vi "CSGaussmeter.setRelvalue.vi"(0 "i ref in":refnum<vi>, 7 "Relative value":dbl, 9 "Unit":T1, 11 "error in (no error)":errorcluster) -> (4 "i ref out":refnum<vi>, 15 "error out":errorcluster)   [LabVIEW 2014, in "CSGaussmeter.lvlib"]
doc: "Dieses VI setzt den Bezugswert für die Relative-Funktion\n\n\nThis VI sets the reference value for the Relative function"
uses:
  CSGaussmeter.lvlib
  instr.lib/FH_55/TypeDef/Unit2.ctl
  CS_Core/CSObj/CSObj.lvlib
  CSlibraries/UtilityLib/UtilityLib.lvlib
  instr.lib/FH_55/FH 55.lvlib
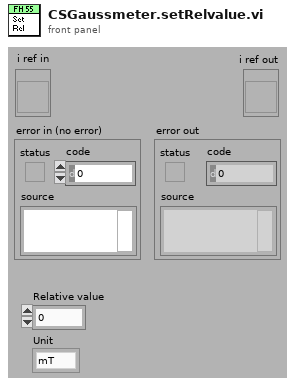
[diagram p1: front panel]
types:
  T1 = typedef "FH 55.lvlib/Unit2.ctl" = enum16{"mT", "G", "kA/m"}
  T2 = typedef "CSGaussmeter.lvlib/CSGaussmeter.i attribute.ctl" = cluster{"Name":string, "VISA Resource Name":refnum<visa-resource-name>, "actValues":cluster{" Limit":bool, "Unit ":T3, "Temp_Unit":T4, "Max":T5, " Filter":bool, " Peak":bool, " Auto_Range":bool, "Range":T6, " Rel":bool, " CTemp":bool, " CField":bool, "AC_DC ":bool, "Set_lower":cluster{"Numeric":dbl, "Cancel Button":bool, "Unit":T1}, "Set_upper":cluster{"Numeric":dbl, "Cancel Button":bool, "Unit":T1}, "Set_Rel":cluster{"Numeric":dbl, "Cancel Button":bool, "Unit":T1}, "Zero":bool, " Local":bool, "Reset":bool, " Init":bool}, "FH 55 Gauss-/Teslameter":T7, "MAX_Value":T8, "MIN_Value":T8, "Rel_Value":T8, "Array ":string[], "LIMU":dbl, " LIML":dbl, "Messwerte 2":string, "Messwerte ":cluster{"Numeric":i32, "OK Button":bool}, "serviceID":cluster{"Current ID":i32, "Unit ID":i32, "Temp ID":i32, "Name ID \n":i32, "Visa ID ":i32}, "setValues ":cluster{" Limit":bool, "Unit ":T3, "Temp_Unit":T4, "Max":T5, " Filter":bool, " Peak":bool, " Auto_Range":bool, "Range":T6, " Rel":bool, " CTemp":bool, " CField":bool, "AC_DC ":bool, "Set_lower":cluster{"Numeric":dbl, "Cancel Button":bool, "Unit":T1}, "Set_upper":cluster{"Numeric":dbl, "Cancel Button":bool, "Unit":T1}, "Set_Rel":cluster{"Numeric":dbl, "Cancel Button":bool, "Unit":T1}, "Zero":bool, " Local":bool, "Reset":bool, " Init":bool}}
  T3 = typedef "FH 55.lvlib/Unit.ctl" = enum16{"T", "G", "A/m"}
  T4 = typedef "FH 55.lvlib/Temp_Unit.ctl" = enum16{"Temp off", "Celsius", "Fahrenheit"}
  T5 = typedef "FH 55.lvlib/Max.ctl" = enum16{"MAX off", "Show MAX", "MAX/MIN"}
  T6 = typedef "FH 55.lvlib/Range.ctl" = enum16{"1", "2", "3", "4", "5", "6", "7"}
  T7 = typedef "FH 55.lvlib/Display.ctl" = cluster{"current value":string, "Limit":string, "Remote":string, "function ":string, "Cluster":cluster{"AC/DC":string, "Auto":string, "Filter":string, "Range":string, "Rel":string, "Peak":string}}
  T8 = typedef "FH 55.lvlib/Value_String.ctl" = cluster{"Numeric":dbl, "String":string}
  T9 = cluster{"Numeric":dbl, "Cancel Button":bool, "Unit":T1}
  T10 = cluster{"VISA Resource Name":refnum<visa-resource-name>}
  T11 = typedef "FH 55.lvlib/VisaCluster.ctl" = cluster{"VISA Resource Name":refnum<visa-resource-name>}
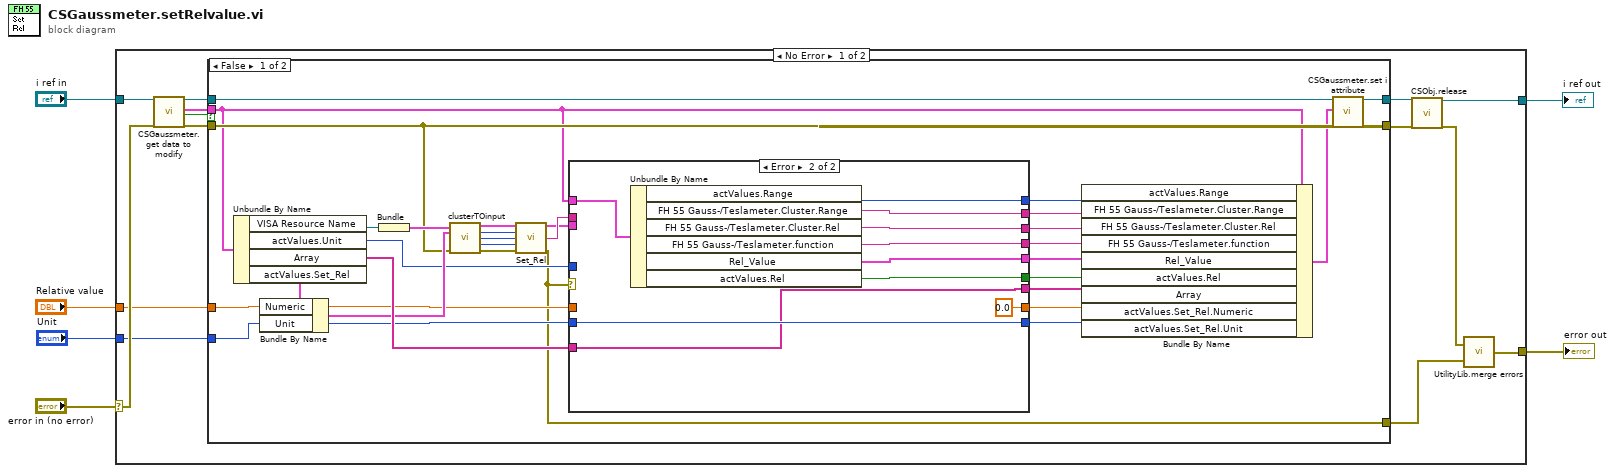
[diagram p0: block diagram]
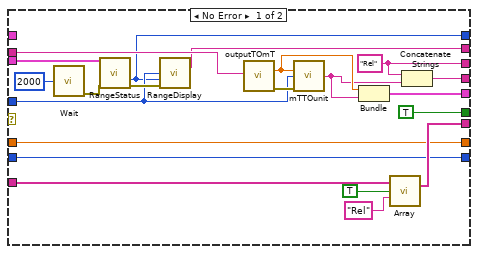
[diagram p2: hidden frame]
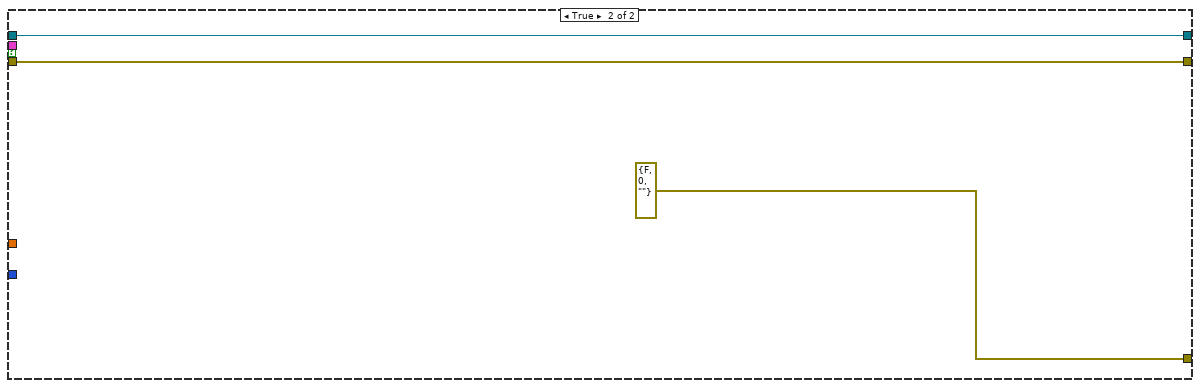
[diagram p3: hidden frame]
diagram:
  n1 = case shown="No Error" "error in (no error)" {
    selector: "error in (no error)" -> [w15 w84]
    tunnel: [w16 w84] -> w3
    tunnel: "i ref in" -> [w14 w85]
    tunnel: [w7 w85] -> w4
    tunnel: "Relative value" -> [w8 _]
    tunnel: "Unit" -> [w9 _]
    frame No Error {
      n2 = call "CSGaussmeter.get data to modify.vi"("i ref in"=w14, "error in (no error)"=w15) -> ("i ref out"=w13:refnum<vi>, "i attribute"=w12:T2, "timed out"=w11:bool, "error out"=w10:errorcluster)  [unwired: 14 in]
      n3 = case shown="False" w11 {
        tunnel: w13 -> [w48 w82]
        tunnel: w10 -> [w32 w83]
        tunnel: w12 -> [w21 _]
        tunnel: [w32 w83] -> w18
        tunnel: [w47 w82] -> w20
        tunnel: [w24 errorcluster {"status"=FALSE, "code"=0, "source"=""} ("error out")] -> w17
        tunnel: w9 -> [w25 _]
        tunnel: w8 -> [w26 _]
        frame False {
          n4 = Unbundle By Name(w21) -> ("VISA Resource Name"=w49:refnum<visa-resource-name>, "actValues.Unit"=w29:T3, "Array"=w39:string[], "actValues.Set_Rel"=w31:T9)
          n5 = Bundle By Name(cluster=w31, "Numeric"=w26, "Unit"=w25) -> (w34:T9)
          n6 = Bundle("VISA Resource Name"=w49) -> (w46:T10)  [unwired: 1 in]
          n7 = call "clusterTOinput.vi"("Set_Rel"=w34, "error in (no error)"=w32) -> ("Range"=w35:T6, "Numeric"=w36:i32, "Unit"=w37:T3, "error out"=w33:errorcluster)  [unwired: 10 in]
          n8 = call "Set_Rel.vi"("VisaCluster"=w46, "Range"=w35, "Numeric"=w36, "Unit"=w37, "error in (no error)"=w33) -> ("VisaCluster"=w30:T11, "Answer"=w43:string, "error out"=w24:errorcluster)  [unwired: 8 in]
          n9 = case shown="Error" w24 {
            tunnel: [TRUE ("actValues.Rel") w72] -> w44
            tunnel: w43 -> [w69 _]
            tunnel: [w68 w74] -> w42
            tunnel: [w67 w73] -> w41
            tunnel: [w66 w71] -> w40
            tunnel: w39 -> [w61 w78]
            tunnel: [w60 w78] -> w38
            tunnel: w30 -> [w58 _]
            tunnel: w29 -> [w56 _]
            tunnel: [w55 w75] -> w28
            tunnel: [w54 w76] -> w27
            tunnel: w26 -> [w53 _]
            tunnel: w25 -> [w52 w80]
            tunnel: [w53 0.0 ("Numeric")] -> w23
            tunnel: [w52 w80] -> w22
            tunnel: w21 -> [_ w77]
            frame No Error {
              w68 = "Rel" ("FH 55 Gauss-/Teslameter.Cluster.Rel")
              n10 = call "Wait.vi"("milliseconds to wait"=u32 2000) -> ("error out"=w51:errorcluster)  [unwired: 14 in]
              n11 = call "RangeStatus.vi"("VisaCluster"=w58, "error in (no error)"=w51) -> ("Range"=w54:T6, "error out"=w57:errorcluster)  [unwired: 10 in, 2 out]
              n12 = call "RangeDisplay.vi"("Unit"=w56, "Range"=w54, "error in (no error)"=w57) -> ("Display"=w55:string)  [unwired: 10 in, 2 out]
              n13 = call "outputTOmT.vi"("Input"=w69) -> ("Numeric"=w65:dbl, "error out"=w59:errorcluster)  [unwired: 13 in]
              n14 = call "mTTOunit.vi"("Numeric"=w65, "Unit"=w56, "error in (no error)"=w59) -> ("Display"=w64:string)  [unwired: 10 in, 2 out]
              n15 = Bundle("Numeric"=w65, "Display"=w64) -> (w66:cluster{"Numeric":dbl, "Display":string})  [unwired: 1 in]
              n16 = call "Array.vi"("Array"=w61, "Boolean"=TRUE, "String"="Rel" ("element")) -> ("Array"=w60:string[])  [unwired: 12 in]
              n17 = Concatenate Strings(w68, w64) -> (w67:string)
            }
            frame Error {
              n18 = Unbundle By Name(w77) -> ("actValues.Range"=w76:T6, "FH 55 Gauss-/Teslameter.Cluster.Range"=w75:string, "FH 55 Gauss-/Teslameter.Cluster.Rel"=w74:string, "FH 55 Gauss-/Teslameter.function"=w73:string, "Rel_Value"=w71:T8, "actValues.Rel"=w72:bool)
            }
          }
          n19 = Bundle By Name(cluster=w21, "actValues.Range"=w27, "FH 55 Gauss-/Teslameter.Cluster.Range"=w28, "FH 55 Gauss-/Teslameter.Cluster.Rel"=w42, "FH 55 Gauss-/Teslameter.function"=w41, "Rel_Value"=w40, "actValues.Rel"=w44, "Array"=w38, "actValues.Set_Rel.Numeric"=w23, "actValues.Set_Rel.Unit"=w22) -> (w45:T2)
          n20 = call "CSGaussmeter.set i attribute.vi"("i ref in"=w48, "i attribute"=w45) -> ("i ref out"=w47:refnum<vi>)  [unwired: 16 in, 1 out]
        }
        frame True {
        }
      }
      n21 = call "CSObj.release.vi"("i ref in"=w20, "error in (no error)"=w18) -> ("i ref out"=w7:refnum<vi>, "error out"=w19:errorcluster)  [unwired: 16 in]
      n22 = call "UtilityLib.merge errors.vi"("error2 (no error)"=w17, "error1 (no error)"=w19) -> ("error out"=w16:errorcluster)
    }
    frame Error {
    }
  }
  "i ref out" <- w4
  "error out" <- w3
